vi "Apply Scale Options GCODE.vi"(6 "Scale Options":T2={"Pos Scale"=1.0, "Vel Scale"=1.0, "G0 Velocity"=100.0, "X Offset"=0.0, "Y Offset"=0.0, "Z Offset"=0.0}, 8 "error in (no error)":errorcluster, 11 "Command Array":T1[](array[typedef])) -> (0 "error out":errorcluster, 3 "Command Array Out":T1[](array[typedef]))   [LabVIEW 2014]
uses:
  Typedefs/GCode Scale Options.ctl
  GCode Parser/GCode Command Cluster.ctl
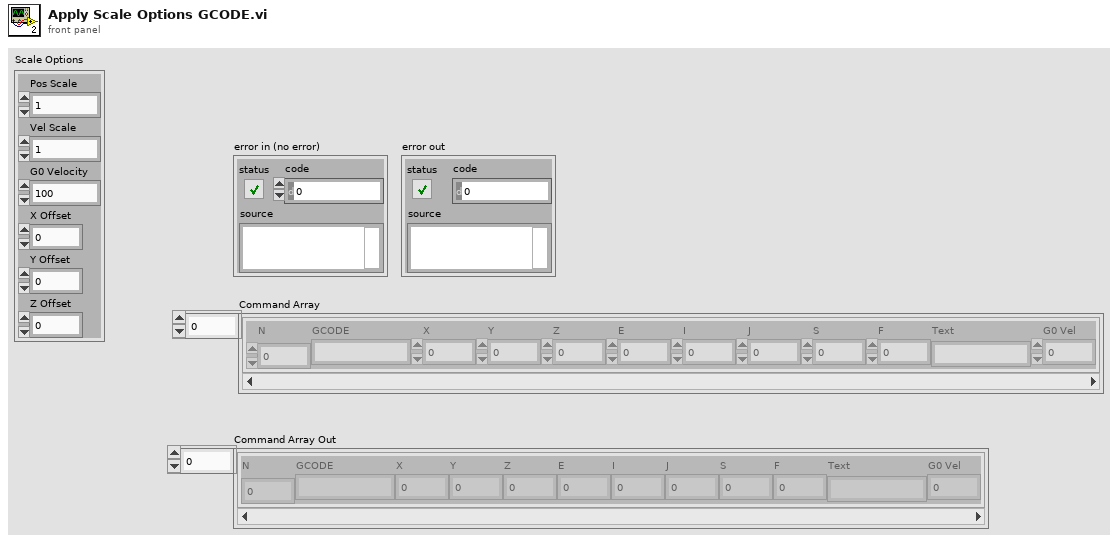
[diagram p1: front panel]
types:
  T1 = typedef "GCode Command Cluster.ctl" = cluster{"N":dbl, "GCODE":string, "X":dbl, "Y":dbl, "Z":dbl, "E":dbl, "I":dbl, "J":dbl, "S":dbl, "F":dbl, "Text":string, "G0 Vel":dbl}
  T2 = typedef "GCode Scale Options.ctl" = cluster{"Pos Scale":dbl, "Vel Scale":dbl, "G0 Velocity":dbl, "X Offset":dbl, "Y Offset":dbl, "Z Offset":dbl}
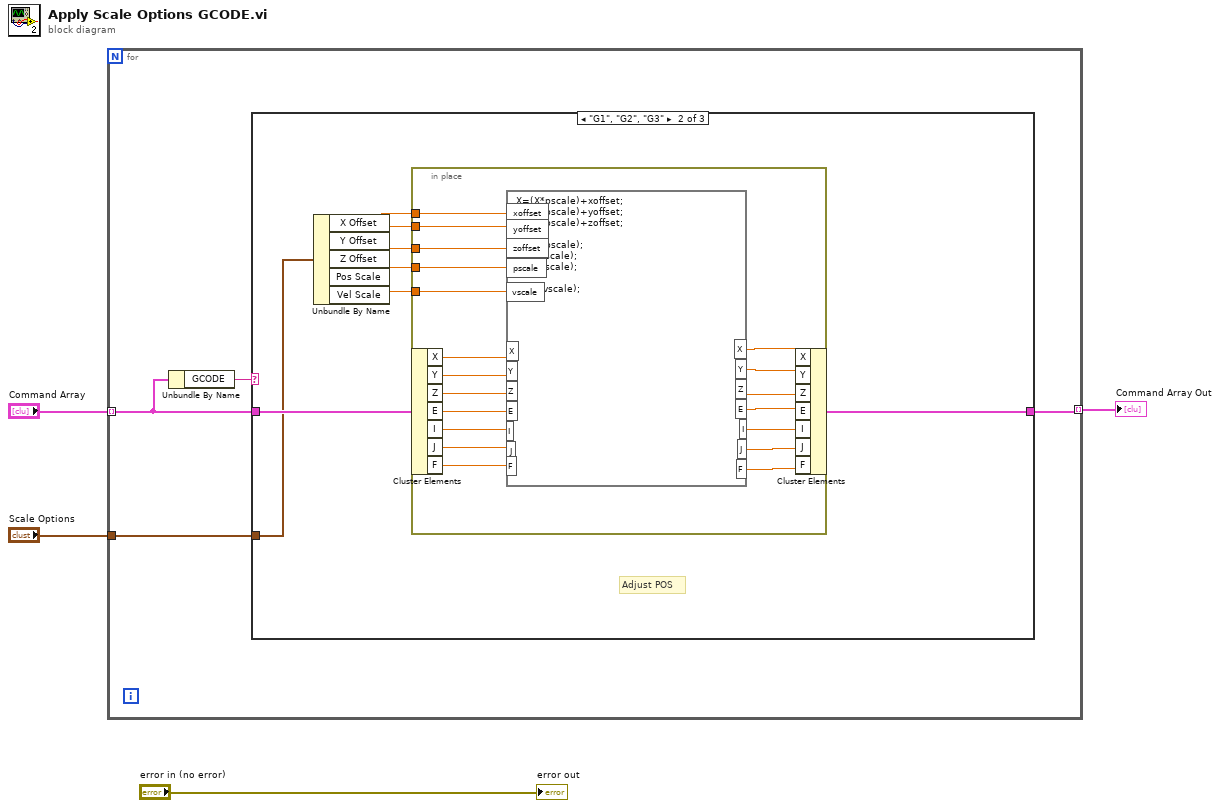
[diagram p0: block diagram]
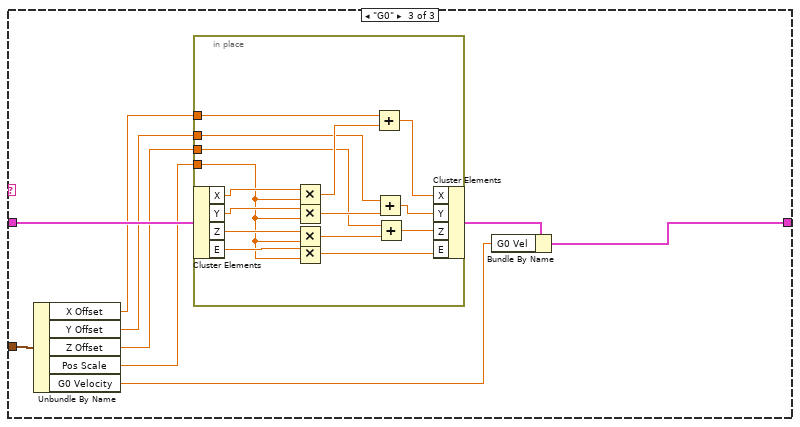
[diagram p3: hidden frame]
diagram:
  n1 = for {
    tunnel: "Scale Options" -> [w7]
    tunnel: "Command Array" -> [w6] mode=indexing
    tunnel: [w5] -> w1 mode=indexing
    n2 = Unbundle By Name(w6) -> ("GCODE"=w8:string)
    n3 = case shown="\"G1\", \"G2\", \"G3\"" w8 {
      tunnel: w6 -> [w9 w17 w45]
      tunnel: [w9 w10 w43] -> w5
      tunnel: w7 -> [_ w16 w42]
      frame "", Default {
      }
      frame "G1", "G2", "G3" {
        # "Adjust POS"
        n4 = Unbundle By Name(w16) -> ("X Offset"=w13:dbl, "Y Offset"=w12:dbl, "Z Offset"=w11:dbl, "Pos Scale"=w15:dbl, "Vel Scale"=w14:dbl)
        n5 = in-place {
          in-place-border: w15 -> [w22]
          in-place-border: w14 -> [w21]
          in-place-border: w13 -> [w20]
          in-place-border: w12 -> [w19]
          in-place-border: w11 -> [w18]
          n6 = in-place-cluster #1(w17) -> ("X"=w36:dbl, "Y"=w35:dbl, "Z"=w30:dbl, "E"=w32:dbl, "I"=w31:dbl, "J"=w34:dbl, "F"=w33:dbl)
          n7 = formula code="X=(X*pscale)+xoffset;\nY=(Y*pscale)+yoffset;\nZ=(Z*pscale)+zoffset;\n\nE=(E*pscale);\nI=(I*pscale);\nJ=(J*pscale);\n\nF=(F*vscale);"("X"=w36, "Y"=w35, "Z"=w30, "E"=w32, "I"=w31, "J"=w34, "pscale"=w22, "vscale"=w21, "xoffset"=w20, "yoffset"=w19, "zoffset"=w18, "F"=w33) -> ("X"=w29:dbl, "Y"=w28:dbl, "Z"=w23:dbl, "E"=w27:dbl, "I"=w26:dbl, "J"=w25:dbl, "F"=w24:dbl)
          n8 = in-place-cluster #1("X"=w29, "Y"=w28, "Z"=w23, "E"=w27, "I"=w26, "J"=w25, "F"=w24) -> (w10:T1)
        }
      }
      frame "G0" {
        n9 = Unbundle By Name(w42) -> ("X Offset"=w39:dbl, "Y Offset"=w38:dbl, "Z Offset"=w37:dbl, "Pos Scale"=w41:dbl, "G0 Velocity"=w40:dbl)
        n10 = in-place {
          in-place-border: w41 -> [w55]
          in-place-border: w39 -> [w52]
          in-place-border: w38 -> [w50]
          in-place-border: w37 -> [w47]
          n11 = in-place-cluster #2(w45) -> ("X"=w60:dbl, "Y"=w59:dbl, "Z"=w58:dbl, "E"=w57:dbl)
          n12 = Multiply(x=w60, y=w55) -> (x*y=w54:dbl)
          n13 = Multiply(x=w59, y=w55) -> (x*y=w49:dbl)
          n14 = Multiply(x=w58, y=w55) -> (x*y=w46:dbl)
          n15 = Multiply(x=w57, y=w55) -> (x*y=w56:dbl)
          n16 = Add(x=w52, y=w54) -> (x+y=w53:dbl)
          n17 = Add(x=w50, y=w49) -> (x+y=w51:dbl)
          n18 = Add(x=w47, y=w46) -> (x+y=w48:dbl)
          n19 = in-place-cluster #2("X"=w53, "Y"=w51, "Z"=w48, "E"=w56) -> (w44:T1)
        }
        n20 = Bundle By Name(cluster=w44, "G0 Vel"=w40) -> (w43:T1)
      }
    }
  }
  "Command Array Out" <- w1
  "error out" <- "error in (no error)"
